vi "Intake Shooter Teleop.vi"(9 "Axes":dbl[](array[numeric]), 11 "Buttons":bool[](array[boolean])) -> ()   [LabVIEW 2019]
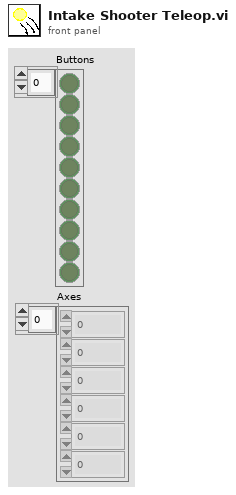
[diagram p1: front panel]
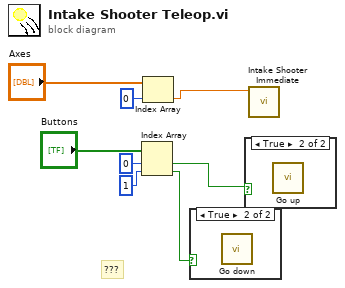
[diagram p0: block diagram]
diagram:
  # "???"
  n1 = Index Array(array="Buttons", index #1=0 ("index"), index #2=1 ("index")) -> (element #1=w2:bool, element #2=w1:bool)
  n2 = Index Array(array="Axes", index=0) -> (element=w3:dbl)
  n3 = case shown="True" w1 {
    frame False {
    }
    frame True {
      n4 = call "Go down.vi"() -> ()  [unwired: 12 in]
    }
  }
  n5 = case shown="True" w2 {
    frame False {
    }
    frame True {
      n6 = call "Go up.vi"() -> ()  [unwired: 12 in]
    }
  }
  n7 = call "Intake Shooter Immediate.vi"("Intake joystick"=w3) -> ()  [unwired: 10 in, 1 out]
